vi "groundwater log header.vi"(0 "NI_report in":refnum<class "NI_report.lvclass">, 5 "error in (no error)":errorcluster, 8 "Groundwater Header":T3, 9 "inside border":T2={"on/off"=TRUE, "weight"=2, "color"=0} {"weight" items=["xlHairline"=1, "xlMedium"=-4138, "xlThick"=4, "xlThin"=2]}, 10 "Worksheet Names":string[](array[string]), 11 "outside border":T2={"on/off"=FALSE, "weight"=2, "color"=0} {"weight" items=["xlHairline"=1, "xlMedium"=-4138, "xlThick"=4, "xlThin"=2]}, 13 "font":T1={"font name"="", "font size"=10.0, "bold"=0, "italic"=0, "underline"=0, "strike through"=0, "font color"=16777216} {"font size" format="%0.2f"; "strike through" items=["Unchanged", "Yes", "No"]; "underline" items=["Unchanged", "Yes", "No"]; "italic" items=["Unchanged", "Yes", "No"]; "bold" items=["Unchanged", "Yes", "No"]}) -> (14 "NI_report out":refnum<class "NI_report.lvclass">, 19 "error out":errorcluster)   [LabVIEW 2016]
uses:
  <vilib>/Utility/NIReport.llb/NI_report.lvclass
  Groundwater header.ctl
  <vilib>/addons/_office/_exclsub.llb/font.ctl
  <vilib>/addons/_office/NI_ReportGenerationToolkit.lvlib
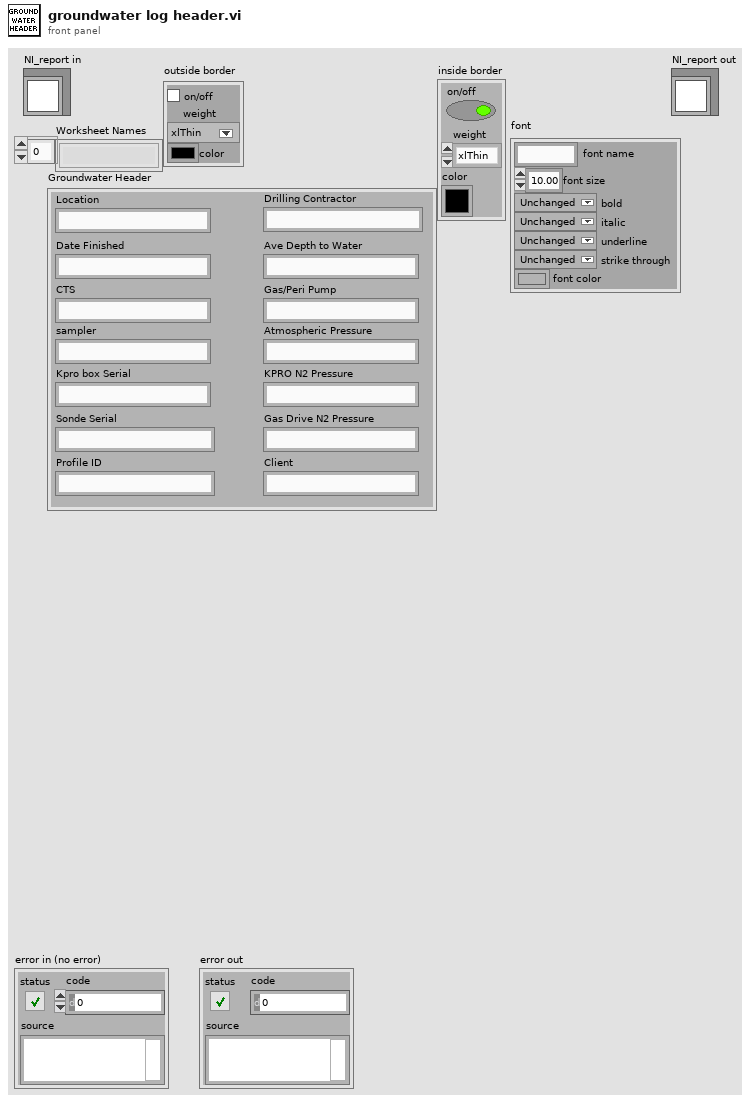
[diagram p1: front panel]
types:
  T1 = typedef "NI_ReportGenerationToolkit.lvlib/font.ctl" = cluster{"font name":string, "font size":dbl, "bold":u16, "italic":u16, "underline":u16, "strike through":u16, "font color":u32}
  T2 = cluster{"on/off":bool, "weight":i32, "color":u32}
  T3 = typedef "Groundwater header.ctl" = cluster{"Location":string, "Date Finished":string, "CTS":string, "sampler":string, "Kpro box Serial ":string, "Sonde Serial":string, "Drilling Contractor":string, "Ave Depth to Water":string, "Gas/Peri Pump":string, "Atmospheric Pressure":string, "KPRO N2 Pressure":string, "Gas Drive N2 Pressure":string, "Profile ID":string, "Client":string}
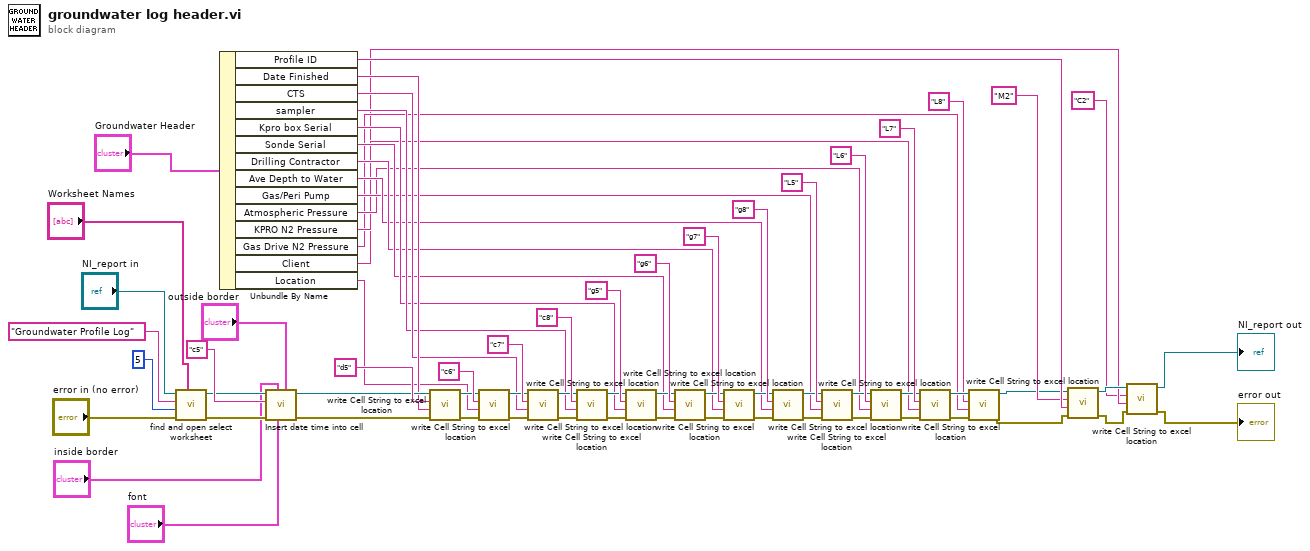
[diagram p0: block diagram]
diagram:
  n1 = call "find and open select worksheet.vi"("Worksheet Names"="Worksheet Names", "error in (no error)"="error in (no error)", "milliseconds to wait"=u32 5, "Worksheet Name in"="Groundwater Profile Log" ("Worksheet Name"), "NI_report in"="NI_report in") -> ("error out"=w32:errorcluster, "NI_report out"=w31:refnum<class "NI_report.lvclass">)  [unwired: 4 in, 1 out]
  n2 = Unbundle By Name("Groundwater Header") -> ("Profile ID"=w14:string, "Date Finished"=w25:string, "CTS"=w24:string, "sampler"=w23:string, "Kpro box Serial"=w22:string, "Sonde Serial"=w21:string, "Drilling Contractor"=w20:string, "Ave Depth to Water"=w19:string, "Gas/Peri Pump"=w18:string, "Atmospheric Pressure"=w17:string, "KPRO N2 Pressure"=w16:string, "Gas Drive N2 Pressure"=w15:string, "Client"=w6:string, "Location"=w1:string)
  n3 = call "Insert date time into cell.vi"("outside border"="outside border", "font"="font", "inside border"="inside border", "error in (no error)"=w32, "Date/Time Cell"="c5", "NI_report in"=w31) -> ("error out"=w35:errorcluster, "NI_report out"=w34:refnum<class "NI_report.lvclass">)  [unwired: 4 in]
  n4 = call "write Cell String to excel location.vi"("error in (no error)"=w35, "input string"=w25, "cell's name"="d5", "NI_report in"=w34) -> ("error out"=w36:errorcluster, "NI_report out"=w37:refnum<class "NI_report.lvclass">)  [unwired: 6 in]
  n5 = call "write Cell String to excel location.vi"("error in (no error)"=w36, "input string"=w1, "cell's name"="c6", "NI_report in"=w37) -> ("error out"=w38:errorcluster, "NI_report out"=w39:refnum<class "NI_report.lvclass">)  [unwired: 6 in]
  n6 = call "write Cell String to excel location.vi"("error in (no error)"=w38, "input string"=w24, "cell's name"="c7", "NI_report in"=w39) -> ("error out"=w40:errorcluster, "NI_report out"=w41:refnum<class "NI_report.lvclass">)  [unwired: 6 in]
  n7 = call "write Cell String to excel location.vi"("error in (no error)"=w40, "input string"=w23, "cell's name"="c8", "NI_report in"=w41) -> ("error out"=w42:errorcluster, "NI_report out"=w44:refnum<class "NI_report.lvclass">)  [unwired: 6 in]
  n8 = call "write Cell String to excel location.vi"("error in (no error)"=w42, "input string"=w22, "cell's name"="g5", "NI_report in"=w44) -> ("error out"=w43:errorcluster, "NI_report out"=w45:refnum<class "NI_report.lvclass">)  [unwired: 6 in]
  n9 = call "write Cell String to excel location.vi"("error in (no error)"=w43, "input string"=w21, "cell's name"="g6", "NI_report in"=w45) -> ("error out"=w53:errorcluster, "NI_report out"=w54:refnum<class "NI_report.lvclass">)  [unwired: 6 in]
  n10 = call "write Cell String to excel location.vi"("error in (no error)"=w53, "input string"=w20, "cell's name"="g7", "NI_report in"=w54) -> ("error out"=w55:errorcluster, "NI_report out"=w56:refnum<class "NI_report.lvclass">)  [unwired: 6 in]
  n11 = call "write Cell String to excel location.vi"("error in (no error)"=w55, "input string"=w19, "cell's name"="g8", "NI_report in"=w56) -> ("error out"=w57:errorcluster, "NI_report out"=w58:refnum<class "NI_report.lvclass">)  [unwired: 6 in]
  n12 = call "write Cell String to excel location.vi"("error in (no error)"=w57, "input string"=w18, "cell's name"="L5", "NI_report in"=w58) -> ("error out"=w61:errorcluster, "NI_report out"=w62:refnum<class "NI_report.lvclass">)  [unwired: 6 in]
  n13 = call "write Cell String to excel location.vi"("error in (no error)"=w61, "input string"=w17, "cell's name"="L6", "NI_report in"=w62) -> ("error out"=w65:errorcluster, "NI_report out"=w66:refnum<class "NI_report.lvclass">)  [unwired: 6 in]
  n14 = call "write Cell String to excel location.vi"("error in (no error)"=w65, "input string"=w16, "cell's name"="L7", "NI_report in"=w66) -> ("error out"=w69:errorcluster, "NI_report out"=w70:refnum<class "NI_report.lvclass">)  [unwired: 6 in]
  n15 = call "write Cell String to excel location.vi"("error in (no error)"=w69, "input string"=w15, "cell's name"="L8", "NI_report in"=w70) -> ("error out"=w12:errorcluster, "NI_report out"=w11:refnum<class "NI_report.lvclass">)  [unwired: 6 in]
  n16 = call "write Cell String to excel location.vi"("error in (no error)"=w12, "input string"=w14, "cell's name"="M2", "NI_report in"=w11) -> ("error out"=w8:errorcluster, "NI_report out"=w10:refnum<class "NI_report.lvclass">)  [unwired: 6 in]
  n17 = call "write Cell String to excel location.vi"("error in (no error)"=w8, "input string"=w6, "cell's name"="C2", "NI_report in"=w10) -> ("error out"=→"error out":errorcluster, "NI_report out"=→"NI_report out":refnum<class "NI_report.lvclass">)  [unwired: 6 in]
